vi "AngleCalc.vi"(1 "Y":dbl, 2 "X":dbl) -> (0 "Angle":dbl)   [LabVIEW 2011]
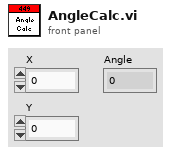
[diagram p1: front panel]
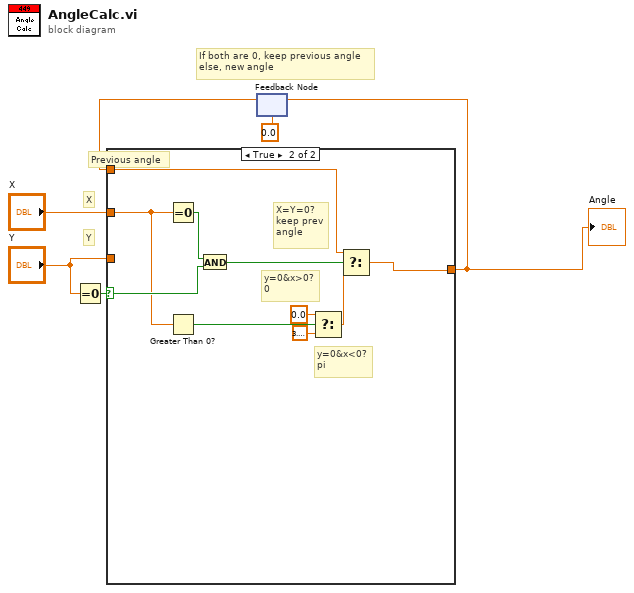
[diagram p0: block diagram]
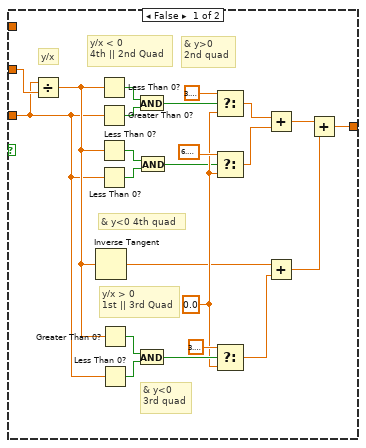
[diagram p2: hidden frame]
diagram:
  # "Previous angle"
  # "X"
  # "Y"
  # "If both are 0, keep previous angle\nelse, new angle"
  n1 = Equal To 0?(x="Y") -> (x = 0?=w4:bool)
  n2 = feedback #1(0.0) -> (w5:dbl)
  n3 = case shown="True" w4 {
    selector: w4 -> [_ w38]
    tunnel: "Y" -> [w7 _]
    tunnel: "X" -> [w29 w30]
    tunnel: [w15 w34] -> w1
    tunnel: w5 -> [_ w33]
    frame False {
      w18 = 0.0 ("f")
      # "& y<0 4th quad"
      # "& y<0\n3rd quad"
      # "& y>0\n2nd quad"
      # "y/x > 0\n1st || 3rd Quad"
      # "y/x < 0\n4th || 2nd Quad"
      # "y/x"
      n4 = Divide(x=w7, y=w29) -> (x/y=w20:dbl)
      n5 = Inverse Tangent(1:w20) -> (0:w12:dbl)
      n6 = Less Than 0?(x=w20) -> (x < 0?=w26:bool)
      n7 = Greater Than 0?(x=w7) -> (x > 0?=w25:bool)
      n8 = Less Than 0?(x=w20) -> (x < 0?=w10:bool)
      n9 = Less Than 0?(x=w7) -> (x < 0?=w9:bool)
      n10 = Greater Than 0?(x=w20) -> (x > 0?=w28:bool)
      n11 = Less Than 0?(x=w7) -> (x < 0?=w27:bool)
      n12 = And(x=w26, y=w25) -> (x .and. y?=w21:bool)
      n13 = And(x=w28, y=w27) -> (x .and. y?=w24:bool)
      n14 = And(x=w10, y=w9) -> (x .and. y?=w8:bool)
      n15 = Select(t=3.141592653589793, s=w21, f=w18) -> (s? t:f=w16:dbl)
      n16 = Select(t=6.283185307179586, s=w8, f=w18) -> (s? t:f=w17:dbl)
      n17 = Select(t=3.141592653589793, s=w24, f=w18) -> (s? t:f=w11:dbl)
      n18 = Add(x=w16, y=w17) -> (x+y=w14:dbl)
      n19 = Add(x=w12, y=w11) -> (x+y=w13:dbl)
      n20 = Add(x=w14, y=w13) -> (x+y=w15:dbl)
    }
    frame True {
      # "y=0&x<0?\npi"
      # "y=0&x>0?\n0"
      # "X=Y=0?\nkeep prev\nangle"
      n21 = Equal To 0?(x=w30) -> (x = 0?=w37:bool)
      n22 = Greater Than 0?(x=w30) -> (x > 0?=w35:bool)
      n23 = And(x=w37, y=w38) -> (x .and. y?=w36:bool)
      n24 = Select(t=0.0, s=w35, f=3.141592653589793) -> (s? t:f=w39:dbl)
      n25 = Select(t=w33, s=w36, f=w39) -> (s? t:f=w34:dbl)
    }
  }
  "Angle" <- w1
  n26 = feedback-in #1(w1) -> ()
